vi "Get Targets_Do.vi"(8 "error in (no error)":errorcluster, 11 "Dependency Source_NIPM in":refnum<class "Dependency Source_NIPM.lvclass">) -> (0 "error out":errorcluster, 1 "Success?":bool, 2 "External Target Map":map{string, string}(c390), 3 "Internal Target Map":map{string, string}(c390), 4 "Unhandled Targets":string[](array[string]))   [LabVIEW 2019, in "Project.Dependencies Finder.lvlib" / "Dependency Source_NIPM.lvclass"]
doc: "Get internal and external targets for the dependency source.\n\nLoads NIPM_External.txt and NIPM_Internal.txt and returns the results. \nNIPM is asked for all packages and the packages found in the files are removed.\n\nFile format is:\n[package name][tab][path1]:[path2]:...\n\nNote: the method of this class will be changed when a better way to find the package paths is found."
uses:
  Dependency Source_NIPM.lvclass
  C:/Current projects/LV32.2019..ProjectDependenciesFinder/Dependency Source/Dependency Source.lvclass
  <vilib>/Utility/sysdir.llb/System Directory Type.ctl
  Project.Dependencies Finder.lvlib
  Dependency Source/Dependency Source.lvclass
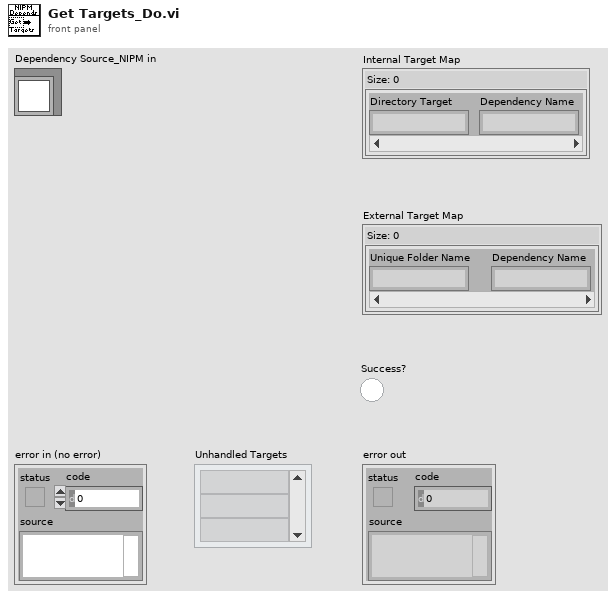
[diagram p1: front panel]
types:
  T1 = typedef "System Directory Type.ctl" = i32
  T2 = cluster{"Path Identifier Array":string[], "Package Name Array":string[]}
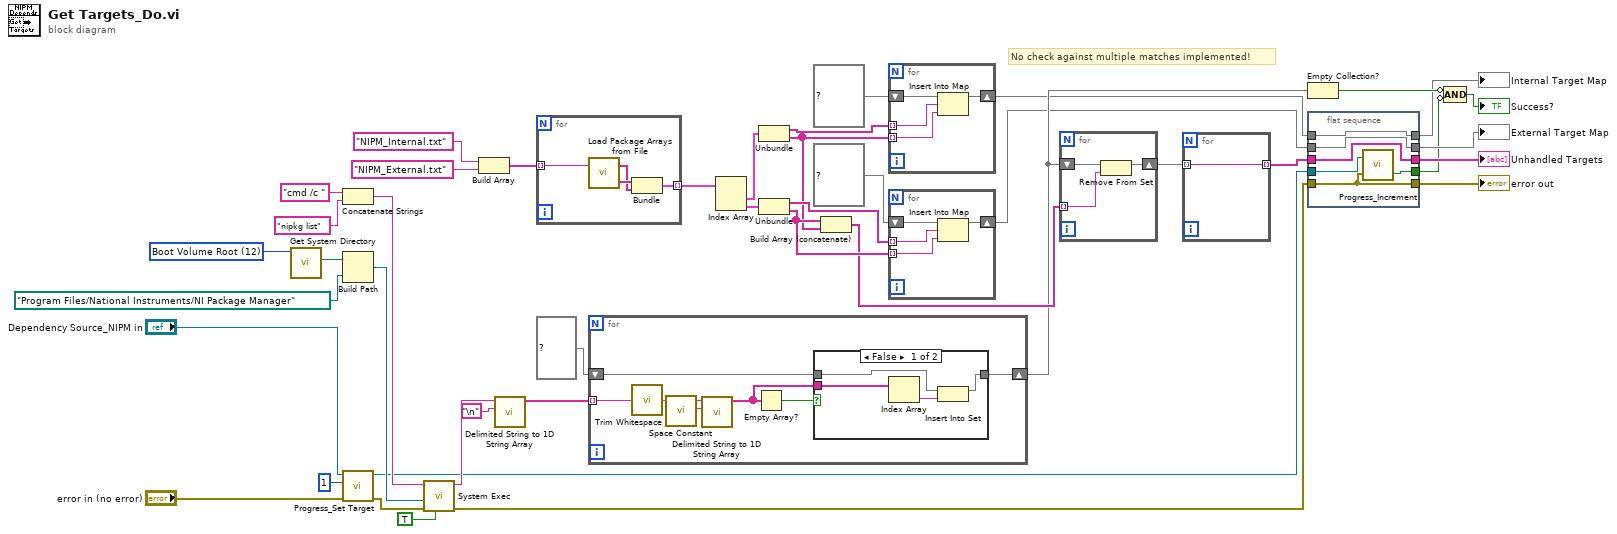
[diagram p0: block diagram]
diagram:
  w30 = T1 12 items=["User Home"=0, "User Desktop"=1, "User Documents"=2, "User Application Data"=3, "User Preferences"=4, "User Temporary"=5, "Public Documents"=6, "Public Application Data"=7, "Public Preferences"=8, "Public Cache"=13, "System Core Libraries"=9, "System Installed Libraries"=10, "Application Files"=11, "Boot Volume Root"=12] ("system directory type")
  # "No check against multiple matches implemented!"
  n1 = call <vilib>:"Get System Directory.vi"("system directory type"=w30) -> ("system directory"=w29:path)  [unwired: 10 in]
  n2 = Concatenate Strings("cmd /c " ("string"), "nipkg list" ("string")) -> (w25:string)
  n3 = Build Path(base path=w29, name or relative path=path "Program Files/National Instruments/NI Package Manager") -> (appended path=w24:path)
  n4 = call "Progress_Set Target.vi"("error in (no error)"="error in (no error)", "Set Target"=1, "Dependency Source in"="Dependency Source_NIPM in") -> ("error out"=w12:errorcluster, "Dependency Source out"=w3:refnum<class "Dependency Source_NIPM.lvclass">)  [unwired: 7 in]
  n5 = call <vilib>:"System Exec.vi"("run minimized? (F)"=TRUE, "error in (no error)"=w12, "working directory"=w24, "command line"=w25) -> ("error out"=w11:errorcluster, "standard output"=w23:string)  [unwired: 4 in, 2 out]
  n6 = Build Array("NIPM_Internal.txt" ("name or relative path"), "NIPM_External.txt" ("name or relative path")) -> (w41:string[])
  n7 = call <vilib>:"Delimited String to 1D String Array.vi"("delimiter"="\n", "delimited string"=w23) -> ("string array"=w21:string[])  [unwired: 9 in]
  n8 = for {
    tunnel: w41 -> [w47] mode=indexing
    tunnel: [w44] -> w40 mode=indexing
    n9 = call "Load Package Arrays from File.vi"("File name"=w47) -> ("Path Identifier Array"=w46:string[], "Package Name Array"=w45:string[])  [unwired: 1 in]
    n10 = Bundle("Path Identifier Array"=w46, "Package Name Array"=w45) -> (w44:T2)  [unwired: 1 in]
  }
  n11 = for {
    tunnel: w21 -> [w54] mode=indexing
    shift-right: [w50] -> w18
    shift-left: set{string} {} ("set") -> [w49]
    n12 = call <vilib>:"Trim Whitespace.vi"("string"=w54) -> ("trimmed string"=w53:string)  [unwired: 1 in]
    n13 = call <vilib>:"Space Constant.vi"() -> ("String"=w52:string)
    n14 = call <vilib>:"Delimited String to 1D String Array.vi"("delimiter"=w52, "delimited string"=w53) -> ("string array"=w48:string[])  [unwired: 9 in]
    n15 = Empty Array?(array=w48) -> (empty?=w51:bool)
    n16 = case shown="False" w51 {
      tunnel: [w57 w59] -> w50
      tunnel: w49 -> [w58 w59]
      tunnel: w48 -> [w56 _]
      frame False {
        n17 = Index Array(array=w56) -> (element=w55:string)  [unwired: 1 in]
        n18 = Insert Into Set(10:w55, 11:w58) -> (3:w57:set{string})  [unwired: 1 out]
      }
      frame True {
      }
    }
  }
  n19 = Index Array(array=w40) -> (element #1=w39:T2, element #2=w38:T2)  [unwired: 2 in]
  n20 = Unbundle(w39) -> ("Path Identifier Array"=w36:string[], "Package Name Array"=w32:string[])
  n21 = Unbundle(w38) -> ("Path Identifier Array"=w35:string[], "Package Name Array"=w33:string[])
  n22 = Build Array (concatenate)(w33, w32) -> (w31:string[])
  n23 = for {
    shift-right: [w62] -> w7
    shift-left: map{string, string} {} ("Internal Target Map") -> [w63]
    tunnel: w36 -> [w61] mode=indexing
    tunnel: w32 -> [w60] mode=indexing
    n24 = Insert Into Map(map in=w63, key=w61, value=w60) -> (map out=w62:map{string, string})  [unwired: 2 out]
  }
  n25 = for {
    shift-right: [w66] -> w5
    shift-left: map{string, string} {} ("External Target Map") -> [w67]
    tunnel: w35 -> [w65] mode=indexing
    tunnel: w33 -> [w64] mode=indexing
    n26 = Insert Into Map(map in=w67, key=w65, value=w64) -> (map out=w66:map{string, string})  [unwired: 2 out]
  }
  n27 = for {
    tunnel: w31 -> [w69] mode=indexing
    shift-right: [w68] -> w19
    shift-left: w18 -> [w70]
    n28 = Remove From Set(10:w69, 11:w70) -> (3:w68:set{string})  [unwired: 1 out]
  }
  n29 = for {
    tunnel: [w71] -> w9 mode=indexing
    tunnel: w19 -> [w71] mode=indexing
  }
  n30 = Empty Collection?(1:w18) -> (0:w17:bool)
  n31 = flat-sequence {
    tunnel: [w74] -> w10
    tunnel: w11 -> [w74]
    tunnel: [w77] -> w8
    tunnel: w9 -> [w77]
    tunnel: w7 -> [w76]
    tunnel: [w76] -> w6
    tunnel: [w75] -> w4
    tunnel: w5 -> [w75]
    tunnel: w3 -> [w73]
    tunnel: [w72] -> w1
    frame #0 {
      n32 = call "Progress_Increment.vi"("error in (sync)"=w74, "Dependency Source in"=w73) -> ("Abort?"=w72:bool)  [unwired: 1 out]
    }
  }
  n33 = Compound Arithmetic op=AND(invert w17, invert w1) -> (→"Success?":bool)
  "error out" <- w10
  "Internal Target Map" <- w6
  "External Target Map" <- w4
  "Unhandled Targets" <- w8
